vi "2 TuningConstants.vi"() -> ()   [LabVIEW 2011]
uses:
  2 Typedefs/PI Constants.ctl
  2 Typedefs/Goodness Weightings.ctl
panel:
  in  "Waypoint Tuning Constant":dbl=80.0 step=0.1
  in  "Wind Adjustment":dbl=0.2 step=0.1
  in  "Goodness Weightings":T1={"Target Importance"=0.98, "No Sail Importance"=1.0, "Change Importance"=0.2, "Pure Waypoint \nImportance"=0.0, "Pure Wind \nImportance"=0.0} {"Pure Wind \nImportance" min=0.0 step=0.2; "Pure Waypoint \nImportance" min=0.0 step=0.2; "Change Importance" min=0.0 step=0.2; "No Sail Importance" min=0.0 step=0.2; "Target Importance" min=0.0 step=0.2}
  in  "No Sail Tuning Quotient":dbl=0.05 step=0.1
  in  "PI Constants":T2={"Proportional Gain"=1.0, "Integral Time"=0.0, "Derivative Time"=0.0}
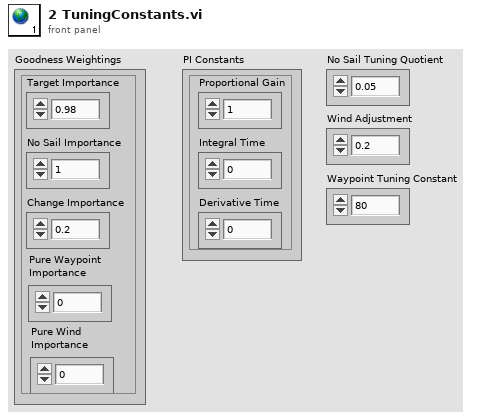
[diagram p1: front panel]
types:
  T1 = typedef "Goodness Weightings.ctl" = cluster{"Target Importance":dbl, "No Sail Importance":dbl, "Change Importance":dbl, "Pure Waypoint \nImportance":dbl, "Pure Wind \nImportance":dbl}
  T2 = typedef "PI Constants.ctl" = cluster{"Proportional Gain":dbl, "Integral Time":dbl, "Derivative Time":dbl}
diagram:
